vi "TEST_L0_MAJ_(3RD)_NEW.vi"(7 "Serial Number":string="SN_test", 8 "error in":errorcluster, 11 "Instrument VISA in":T1={"AWG VISA"="AgilentGen1", "Oscilloscope  VISA "="AgilentOsc", "Integration Board IP"="172.16.17.47", "connection ID"=refnum, "report out"=refnum, "report file path"=path "C:/Users/omartinez/Desktop/L0nL1_Results"}) -> (0 "error out":errorcluster, 3 "Instrument VISA out":T1={"AWG VISA"="AgilentGen1", "Oscilloscope  VISA "="AgilentOsc", "Integration Board IP"="172.16.17.47", "connection ID"=refnum, "report out"=refnum, "report file path"=path "C:/Users/omartinez/Desktop/L0nL1_Results"}, 5 "ThresholdOut":i32[][](array[numeric])=[[518, 524, 524, 522, 522, 514, 510], [522, 526, 528, 526, 524, 518, 514], [530, 536, 534, 532, 530, 524, 524], [552, 550, 520, 518, 558, 546, 544], [584, 590, 582, 590, 586, 570, 578]])   [LabVIEW 2012]
uses:
  <vilib>/Utility/NIReport.llb/NI_report.lvclass
  <vilib>/Utility/NIReport.llb/HTML/NI_HTML.lvclass
  <instrlib>/Agilent 8000 Series/Public/Configure/Configure Math (Binary Operation).vi
  Sum_Abrilader/L0_Sum_Adder Folder/C/Program Files/National Instruments/LabVIEW 2012/instr.lib/Agilent 8000 Series/Public/Data/Low Level/Fetch Measurement (More).vi
  <instrlib>/Agilent 8000 Series/Agilent 8000 Series.lvlib
panel:
  in  "Att gain":u32=15
  out "IPR_count":u32
  in  "Threshold Limits":i32[](array[numeric])=[500, 1024]
  in  "Voltages comprobation":dbl[](array[numeric])=[0.05, 0.1, 0.2, 0.5, 0.8]
  in  "Channels":i32[](array[numeric])=[0, 1, 2, 3, 4, 5, 6]
  out "threshold out":i32=564
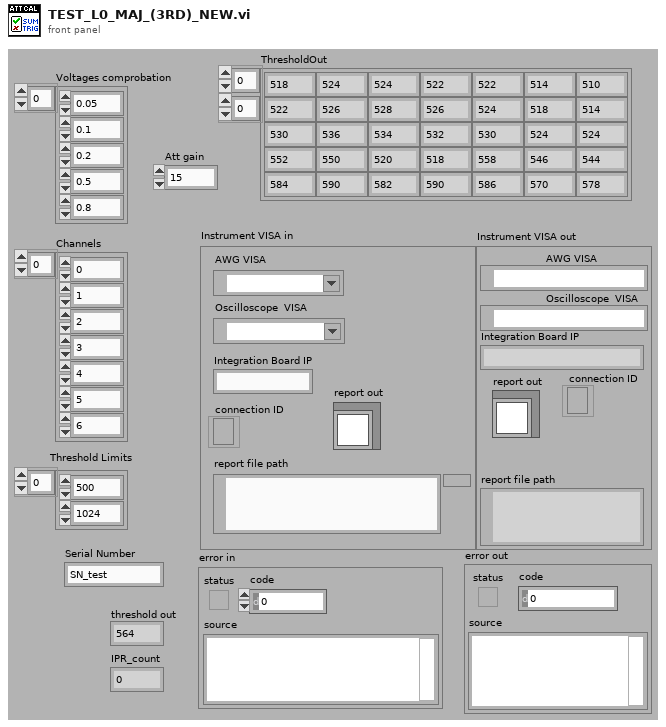
[diagram p1: front panel]
types:
  T1 = cluster{"AWG VISA":refnum<visa-resource-name>, "Oscilloscope  VISA ":refnum<visa-resource-name>, "Integration Board IP":string, "connection ID":refnum<k5>, "report out":refnum<class "NI_report.lvclass">, "report file path":path}
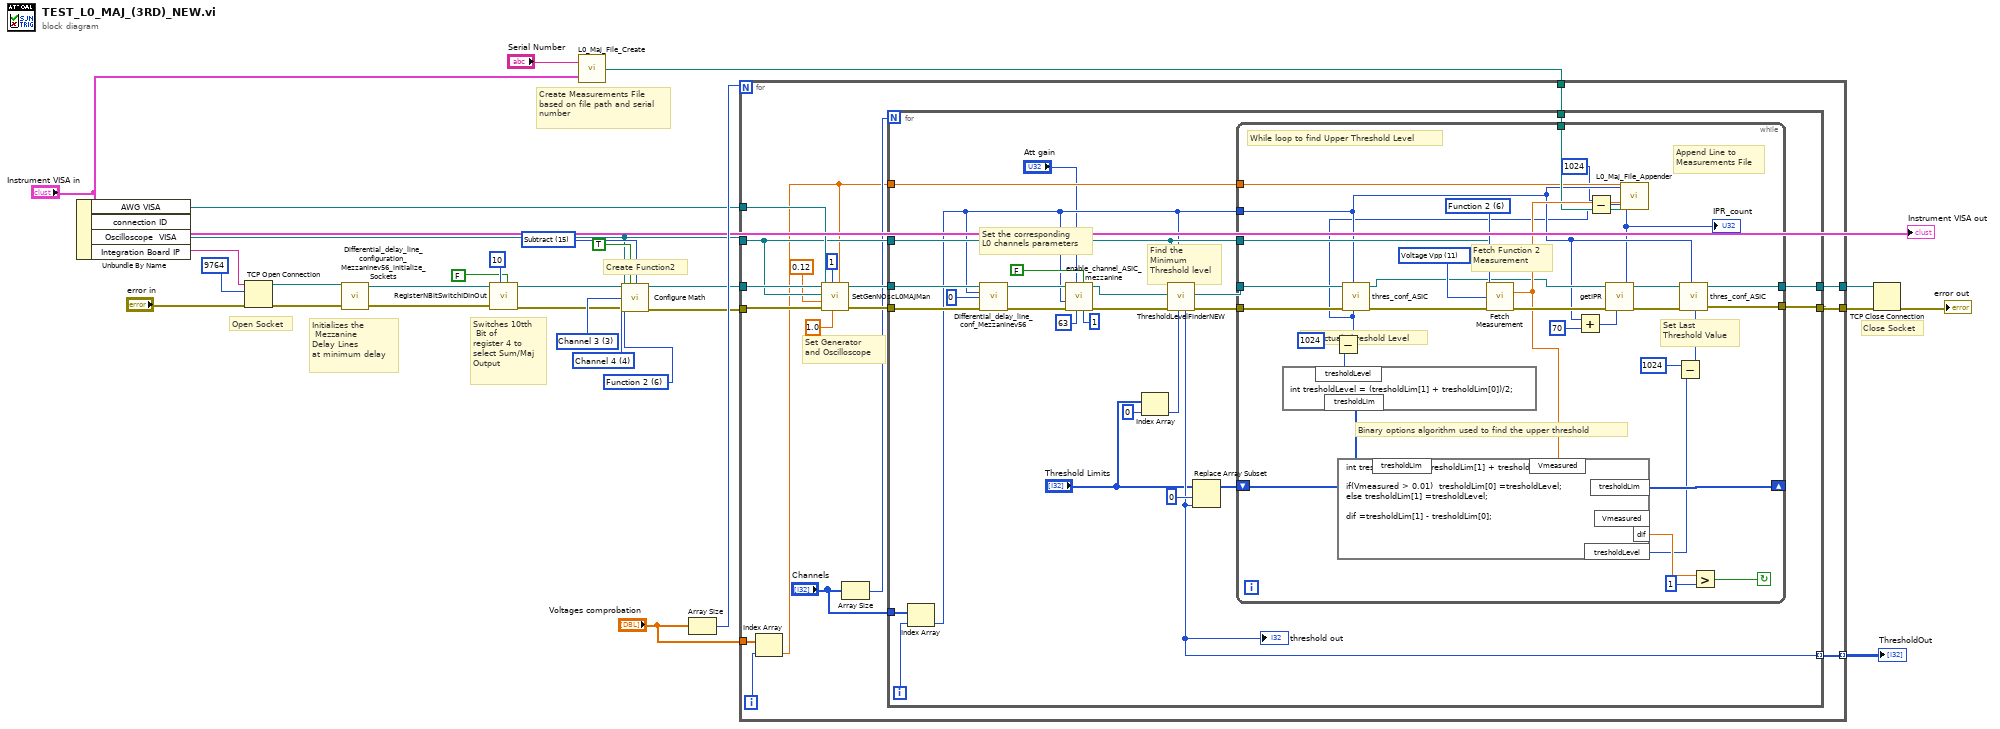
[diagram p0: block diagram]
diagram:
  w14 = u16 6 items=["Function 1"=5, "Function 2"=6, "Function 3"=7, "Function 4"=8] ("Math Channel (5: Function 1)")
  w15 = u16 15 items=["Add"=12, "Divide"=13, "Multiply"=14, "Subtract"=15, "Common Mode"=16, "Versus"=17] ("Math Operation (12: Add)")
  w13 = 3 items=["Channel 1"=1, "Channel 2"=2, "Channel 3"=3, "Channel 4"=4] ("Channel (1: Channel 1)")
  w12 = 4 items=["Channel 1"=1, "Channel 2"=2, "Channel 3"=3, "Channel 4"=4] ("Channel (1: Channel 1)")
  # "Initializes the\n Mezzanine\nDelay Lines \nat minimum delay"
  # "Switches 10tth \n Bit of\nregister 4 to \nselect Sum/Maj\nOutput"
  # "Close Socket"
  # "Create Function2"
  # "Open Socket"
  # "Create Measurements File\nbased on file path and serial\nnumber"
  n1 = Unbundle By Name("Instrument VISA in") -> ("AWG VISA"=w9:refnum<visa-resource-name>, "Oscilloscope  VISA"=w10:refnum<visa-resource-name>, "Integration Board IP"=w24:string)  [unwired: 1 out]
  n2 = TCP Open Connection(address=w24, remote port or service name=u16 9764, error in (no error)="error in") -> (connection ID=w3:refnum<k5>, error out=w5:errorcluster)  [unwired: 2 in]
  n3 = call "Differential_delay_line_configuration_Mezzaninev56_initialize_Sockets.vi"("connection ID"=w3, "error in (no error)"=w5) -> ("connection ID out"=w6:refnum<k5>, "error out 2"=w7:errorcluster)  [unwired: 6 in]
  n4 = call "RegisterNBitSwitchIDInOut.vi"("Switch Bit"=FALSE, "N Bit"=10, "error in (no error)"=w7, "connection ID"=w6) -> ("error out"=w4:errorcluster, "connection ID out"=w2:refnum<k5>)  [unwired: 5 in]
  n5 = call "L0_Maj_File_Create.vi"("input cluster"="Instrument VISA in", "Serial Number"="Serial Number") -> ("appended path"=w17:path)
  n6 = call-poly <instrlib>:"Configure Math.vi"("VISA resource name"=w10, "Enable Math Channel (T:Enable)"=TRUE, "Math Operation (12: Add)"=w15, "Math Channel (5: Function 1)"=w14, "Math Operand (1: Channel 1)"=w13, "Math Operand (2: Channel 2)"=w12, "error in (no error)"=w4) -> ("error out"=w11:errorcluster)  [unwired: 7 in, 1 out]
  n7 = Array Size(array="Voltages comprobation") -> (size(s)=w22:i32)
  n8 = for {
    N: w22 -> [_]
    tunnel: [w45] -> w26
    tunnel: [w44] -> w25
    tunnel: w11 -> [w38]
    tunnel: w2 -> [w37]
    tunnel: w10 -> [w35]
    tunnel: w9 -> [w39]
    tunnel: "Voltages comprobation" -> [w43]
    tunnel: [w32] -> w20 mode=indexing
    tunnel: w17 -> [w31]
    i -> [w42]
    # "Set Generator\nand Oscilloscope"
    n9 = Index Array(array=w43, index=w42) -> (element=w29:dbl)
    n10 = call "SetGenNOscL0MAJMan.vi"("Input Voltage"=w29, "Amp Scaler"=1.0, "NChannels"=1, "error in (no error)"=w38, "Output Voltage"=0.12 ("Input Voltage"), "VISA resource name"=w35, "AWG VISA"=w39) -> ("error out 2"=w36:errorcluster)  [unwired: 4 in]
    n11 = Array Size(array="Channels") -> (size(s)=w34:i32)
    n12 = for {
      N: w34 -> [_]
      tunnel: [w59] -> w45
      tunnel: [w60] -> w44
      tunnel: w37 -> [w64]
      tunnel: w36 -> [w63]
      tunnel: w35 -> [w56]
      tunnel: "Channels" -> [w62]
      tunnel: [w53] -> w32 mode=indexing
      tunnel: w31 -> [w51]
      tunnel: w29 -> [w50]
      i -> [w61]
      # "Find the\nMinimum \nThreshold level"
      # "Set the corresponding\nL0 channels parameters"
      n13 = Index Array(array=w62, index=w61) -> (element=w55:i32)
      n14 = call "Differential_delay_line_conf_Mezzaninev56.vi"("connection ID"=w64, "channel"=w55, "Delay value"=u16 0, "error in (no error)"=w63) -> ("connection ID out"=w70:refnum<k5>, "error out 2"=w71:errorcluster)  [unwired: 4 in, 6 out]
      n15 = call "enable_channel_ASIC_mezzanine.vi"("Clip_sel_b"=u32 1, "maj/sum"=FALSE, "Ib_clipVb"=u32 63, "Att gain"="Att gain", "error in"=w71, "Channel"=w55, "connection ID"=w70) -> ("error out"=w65:errorcluster, "connection ID out"=w66:refnum<k5>)  [unwired: 2 in, 1 out]
      n16 = Index Array(array="Threshold Limits", index=0) -> (element=w47:i32)
      n17 = call "ThresholdLevelFinderNEW.vi"("Initial Threshold"=w47, "Channel"=w55, "error in (no error)"=w65, "connection ID"=w66, "VISA resource name"=w56) -> ("error out"=w58:errorcluster, "connection ID out"=w57:refnum<k5>, "threshold out"=w53:i32)  [unwired: 2 in, 2 out]
      "threshold out" <- w53
      n18 = Replace Array Subset(array="Threshold Limits", new element=w53, index=u32 0 ("Att gain")) -> (w52:i32[])
      n19 = while {
        tunnel: [w104] -> w60
        tunnel: [w79] -> w59
        tunnel: w58 -> [w103]
        tunnel: w57 -> [w102]
        tunnel: w56 -> [w99]
        tunnel: w55 -> [w82]
        shift-right: [w92] -> _
        shift-left: w52 -> [w91]
        tunnel: w51 -> [w89]
        tunnel: w50 -> [w88]
        stop <- w95 continue-if-true
        w101 = 11 items=["Rise Time", "Fall Time", "Frequency", "Period", "Voltage RMS(AC)", "Voltage RMS(DC)", "Voltage RMS (AC,cycle)", "Voltage RMS (DC,cycle)", "Voltage Max", "Voltage Min", "Voltage Middle", "Voltage Vpp", "Voltage High", "Voltage Low", "Voltage Average", "Voltage Average (cycle)", "Width Negative", "Width Positive", "Duty Cycle Positive", "Amplitude", "Overshoot", "Preshoot", "Voltage Base", "Voltage Upper", "Time Max", "Time Min", "Color Grade Crossing", "Color Grade Eye Width", "Color Grade Eye Height", "Color Grade Eye Q-Factory", "Color Grade Eye Duty Cycle Distortion(Percent)", "Color Grade Eye Duty Cycle Distortion(Time)", "Color Grade Eye Jitter(PP)", "Color Grade Eye Width(RMS)", "Cycle-cycle Duty Jitter(Rising)", "Cycle-cycle Duty Jitter(Falling)", "Cycle-cycle Jitter(Rising)", "Cycle-cycle Jitter(Falling)", "Cycle-cycle - Width", "Cycle-cycle + Width", "Date Rate", "Unit Interval", "FFT Delta Frequency", "FFT Delta Magnitude", "FFT Frequency", "FFT Magnitude", "Slew Rate", "Area (Entire Display)", "Area(Single Cycle)", "Duty Cycle (Rising)", "Duty Cycle (Falling)"] ("Measurement Function (0: Rise Time)")
        w100 = 6 items=["Channel 1"=1, "Channel 2"=2, "Channel 3"=3, "Channel 4"=4, "Function 1"=5, "Function 2"=6, "Function 3"=7, "Function 4"=8, "Memory 1"=9, "Memory 2"=10, "Memory 3"=11, "Memory 4"=12] ("Channel (1: Channel 1)")
        # "Binary options algorithm used to find the upper threshold"
        # "Set Last \nThreshold Value"
        # "While loop to find Upper Threshold Level"
        # "Set Actual Threshold Level"
        # "Append Line to \nMeasurements File"
        # "Fetch Function 2\nMeasurement"
        n20 = formula code="int tresholdLevel = (tresholdLim[1] + tresholdLim[0])/2;"("tresholdLim"=w91) -> ("tresholdLevel"=w87:i32)
        n21 = Subtract(x=1024, y=w87) -> (x-y=w73:i32)
        n22 = call "thres_conf_ASIC.vi"("threshold"=w73, "Ring"=w82, "error out 3"=w103, "connection ID"=w102) -> ("error out 2"=w98:errorcluster, "connection ID out"=w85:refnum<k5>)  [unwired: 4 in, 2 out]
        n23 = call-poly "Fetch Measurement.vi"("VISA resource name"=w99, "Channel (1: Channel 1)"=w100, "Measurement Function (0: Rise Time)"=w101, "error in (no error)"=w98) -> ("Measurement"=w93:dbl, "error out"=w97:errorcluster)  [unwired: 9 in, 1 out]
        n24 = formula code="int tresholdLevel = (tresholdLim[1] + tresholdLim[0])/2;\n\nif(Vmeasured > 0.01)  tresholdLim[0] =tresholdLevel;\nelse tresholdLim[1] =tresholdLevel;\n\ndif =tresholdLim[1] - tresholdLim[0];"("Vmeasured"=w93, "tresholdLim"=w91) -> ("dif"=w94:dbl, "tresholdLevel"=w90:i32, "tresholdLim"=w92:i32[])  [unwired: 1 out]
        n25 = Add(x=w82, y=70) -> (x+y=w81:i32)
        n26 = Subtract(x=1024 ("x-y"), y=w73) -> (x-y=w75:i32)
        n27 = call "getIPR.vi"("Address"=w81, "error in"=w97, "connection ID"=w85) -> ("error out"=w86:errorcluster, "connection ID out"=w84:refnum<k5>, "IPR_count"=w80:u32)  [unwired: 5 in, 1 out]
        "IPR_count" <- w80
        n28 = call "L0_Maj_File_Appender.vi"("Vin"=w88, "CH"=w82, "Vmeas"=w93, "Threshold"=w75, "file path (dialog if empty)"=w89, "DT"=w80) -> ()  [unwired: 22 in]
        n29 = Subtract(x=1024, y=w90) -> (x-y=w77:i32)
        n30 = call "thres_conf_ASIC.vi"("threshold"=w77, "Ring"=w82, "error out 3"=w86, "connection ID"=w84) -> ("error out 2"=w79:errorcluster, "connection ID out"=w104:refnum<k5>)  [unwired: 4 in, 2 out]
        n31 = Greater?(x=w94, y=1) -> (0:w95:bool)
      }
    }
  }
  "ThresholdOut" <- w20
  n32 = TCP Close Connection(connection ID=w25, error in (no error)=w26) -> (error out=→"error out":errorcluster)  [unwired: 1 in, 1 out]
  "Instrument VISA out" <- "Instrument VISA in"
